vi "Remove Raw XML Tag from Data Name.vi"(11 "Data Name":string) -> (2 "Data Name without #xml":string, 3 "Raw XML?":bool)   [LabVIEW 2013]
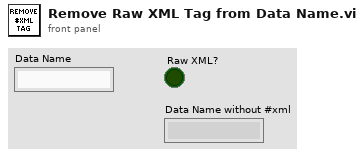
[diagram p1: front panel]
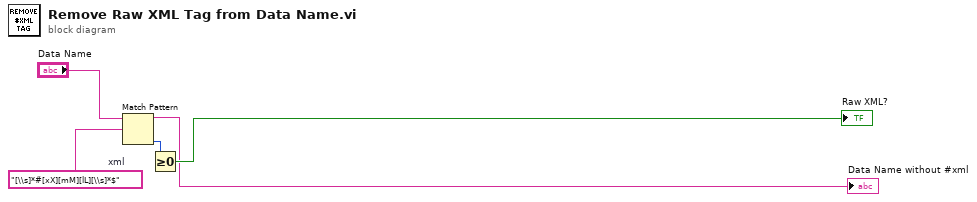
[diagram p0: block diagram]
diagram:
  w1 = "[\\s]*#[xX][mM][lL][\\s]*$"  # xml
  n1 = Match Pattern(string="Data Name", regular expression=w1) -> (before substring=→"Data Name without #xml":string, offset past match=w4:i32)  [unwired: 1 in, 2 out]
  n2 = Greater Or Equal To 0?(x=w4) -> (x >= 0?=→"Raw XML?":bool)
